vi "Convert A to T.vi"(7 "PS Model Cluster":T1, 8 "LTS Slew [A/S] in":dbl, 9 "LTS Setpoint [A] in":dbl, 10 "HTS Slew [A/S] in":dbl, 11 "HTS Setpoint [A] in":dbl) -> (0 "LTS Slew [A/S] out":dbl, 1 "LTS Setpoint [A] out":dbl, 2 "HTS Slew [A/S] out":dbl, 3 "HTS Setpoint [A] out":dbl)   [LabVIEW 2023]
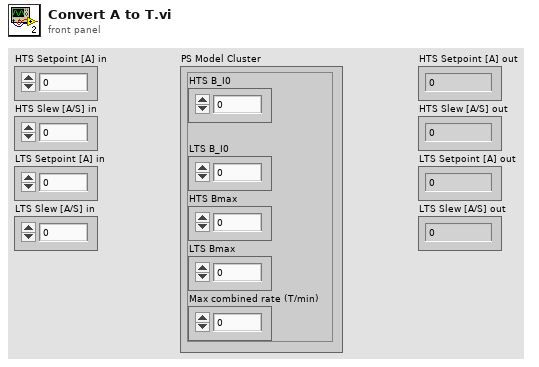
[diagram p1: front panel]
types:
  T1 = cluster{"HTS B_I0":dbl, "LTS B_I0":dbl, "HTS Bmax":dbl, "LTS Bmax":dbl, "Max combined rate (T/min)":dbl}
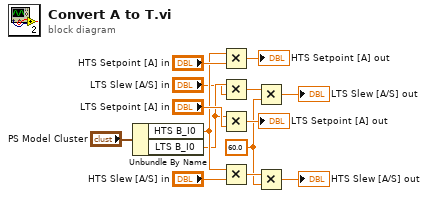
[diagram p0: block diagram]
diagram:
  w3 = 60.0 ("y")
  n1 = Unbundle By Name("PS Model Cluster") -> ("HTS B_I0"=w9:dbl, "LTS B_I0"=w8:dbl)
  n2 = Multiply(x=w9, y="HTS Setpoint [A] in") -> (x*y=→"HTS Setpoint [A] out":dbl)
  n3 = Multiply(x=w8, y="LTS Slew [A/S] in") -> (x*y=w4:dbl)
  n4 = Multiply(x=w8, y="LTS Setpoint [A] in") -> (x*y=→"LTS Setpoint [A] out":dbl)
  n5 = Multiply(x=w9, y="HTS Slew [A/S] in") -> (x*y=w5:dbl)
  n6 = Multiply(x=w4, y=w3) -> (x*y=→"LTS Slew [A/S] out":dbl)
  n7 = Multiply(x=w5, y=w3) -> (x*y=→"HTS Slew [A/S] out":dbl)
